vi "读取状态值.vi"(8 "error in (no error)":errorcluster, 10 "Slave ID":u8=1, 11 "MB session in":refnum<class "MB_Master.lvclass">) -> (0 "error out":errorcluster, 1 "Registers":u16[](array[numeric]), 2 "状态值":T1, 3 "MB session out":refnum<class "MB_Master.lvclass">)   [LabVIEW 2016, in "流量计集成.lvlib" / "斯坦道功率测流.lvlib"]
uses:
  <vilib>/Plasmionique/MB Master/MB_Master/MB_Master.lvclass
  <vilib>/Plasmionique/MB Master/MB Master.lvlib
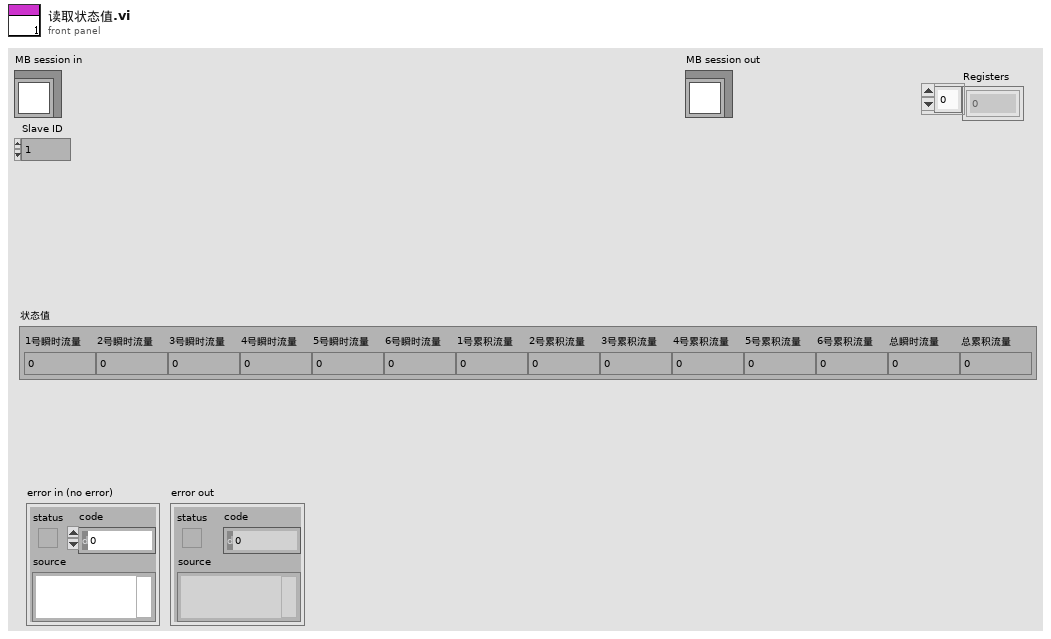
[diagram p1: front panel]
types:
  T1 = typedef "流量计集成.lvlib/斯坦道功率测流.lvlib/状态值.ctl" = cluster{"1号瞬时流量":dbl, "2号瞬时流量":dbl, "3号瞬时流量":dbl, "4号瞬时流量":dbl, "5号瞬时流量":dbl, "6号瞬时流量":dbl, "1号累积流量":dbl, "2号累积流量":dbl, "3号累积流量":dbl, "4号累积流量":dbl, "5号累积流量":dbl, "6号累积流量":dbl, "总瞬时流量":dbl, "总累积流量":dbl}
  T2 = cluster{"CDAB[0]":sgl, "CDAB[1]":sgl, "CDAB[2]":sgl, "CDAB[3]":sgl, "CDAB[4]":sgl, "CDAB[5]":sgl, "CDAB[6]":sgl, "CDAB[7]":sgl, "CDAB[8]":sgl, "CDAB[9]":sgl, "CDAB[10]":sgl, "CDAB[11]":sgl, "CDAB[12]":sgl, "CDAB[13]":sgl}
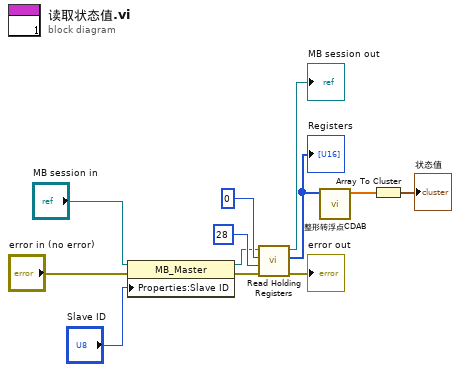
[diagram p0: block diagram]
diagram:
  n1 = property class="MB_Master"(reference="MB session in", error in="error in (no error)", "Properties:Slave ID"="Slave ID") -> (reference out=w7:refnum<class "MB_Master.lvclass">, error out=w5:errorcluster)
  n2 = call <vilib>:"Read Holding Registers.vi"("error in (no error)"=w5, "quantity"=u16 28, "starting address"=u16 0, "MB session in"=w7) -> ("error out"=→"error out":errorcluster, "Registers"=w3:u16[], "MB session out"=→"MB session out":refnum<class "MB_Master.lvclass">)  [unwired: 5 in]
  "Registers" <- w3
  n3 = call "整形转浮点CDAB.vi"("数组"=w3) -> ("CDAB"=w2:sgl[])  [unwired: 10 in]
  n4 = Array To Cluster(array=w2) -> (cluster=→"状态值":T2)
